vi "tm484_highcontrastmode.vi"() -> ()   [LabVIEW 2019]
panel:
  in  "High Contrast":bool
  out "Timestamp":dbl
  out "DCAM Version":string
  out "Library Version":string
  out "Image":u16[][](graph)
  out "Frames Per Second":dbl
  in  "Quit":bool
  out "Error Out":errorcluster {"code" format="%.0x"}
  # "This is just a simple example\nof how to capture and display\nlive data."
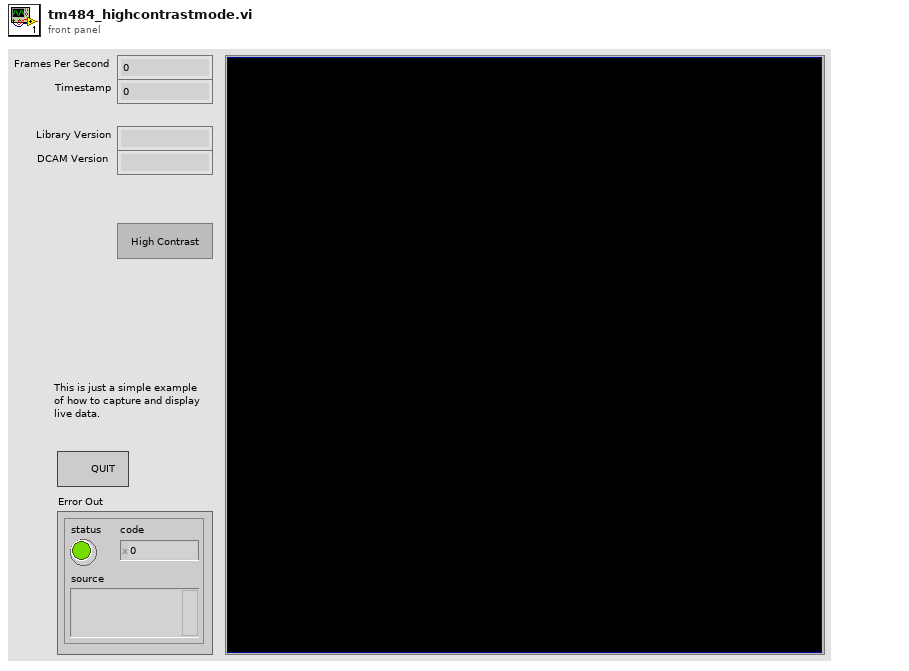
[diagram p1: front panel]
types:
  T1 = cluster{"Capture Library":string, "DCAM-API":string}
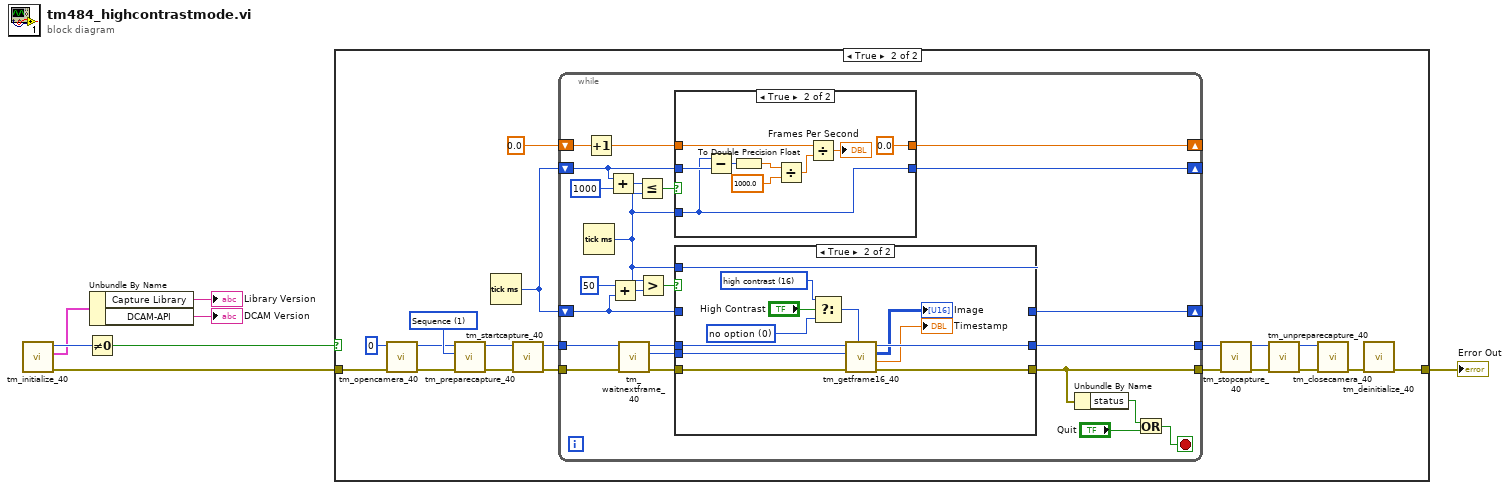
[diagram p0: block diagram]
diagram:
  n1 = call <userlib>:"tm_initialize_40.vi"() -> ("error out"=w4:errorcluster, "Version Info"=w3:T1, "Number Of Cameras"=w5:u32)  [unwired: 8 in, 1 out]
  n2 = Not Equal To 0?(x=w5) -> (x != 0?=w7:bool)
  n3 = Unbundle By Name(w3) -> ("Capture Library"=→"Library Version":string, "DCAM-API"=→"DCAM Version":string)
  n4 = case shown="True" w7 {
    tunnel: w4 -> [w8 w27]
    tunnel: [w8 w24] -> w6
    frame False {
    }
    frame True {
      w15 = 1 items=["Snap", "Sequence"] ("Capture mode")
      n5 = call <userlib>:"tm_opencamera_40.vi"("error in (no error)"=w27, "Camera Index"=u32 0) -> ("error out"=w9:errorcluster, "Handle out"=w10:u32)  [unwired: 7 in, 1 out]
      n6 = call <userlib>:"tm_preparecapture_40.vi"("error in (no error)"=w9, "Capture mode"=w15, "Handle in"=w10) -> ("error out"=w13:errorcluster, "Handle out"=w14:u32)  [unwired: 5 in, 2 out]
      n7 = Tick Count (ms)() -> (millisecond timer value=w11:u32)
      n8 = call <userlib>:"tm_startcapture_40.vi"("error in (no error)"=w13, "Handle in"=w14) -> ("error out"=w16:errorcluster, "Handle out"=w17:u32)  [unwired: 8 in]
      n9 = while {
        tunnel: [w30] -> w20
        tunnel: [w31] -> w21
        tunnel: w17 -> [w48]
        tunnel: w16 -> [w49]
        shift-right: [w46] -> _
        shift-left: w11 -> [w43]
        shift-right: [w47] -> _
        shift-left: 0.0 -> [w40]
        shift-right: [w29] -> _
        shift-left: w11 -> [w32]
        stop <- w28 stop-if-true
        n10 = Tick Count (ms)() -> (millisecond timer value=w33:u32)
        n11 = Increment(x=w40) -> (x+1=w41:dbl)
        n12 = Add(x=w43, y=u32 1000) -> (x+y=w45:u32)
        n13 = Add(x=u32 50, y=w32) -> (x+y=w35:u32)
        n14 = call <userlib>:"tm_waitnextframe_40.vi"("error in (no error)"=w49, "Handle in"=w48) -> ("error out"=w38:errorcluster, "Frame Index"=w37:i32, "Handle out"=w39:u32)  [unwired: 6 in, 1 out]
        n15 = Less Or Equal?(x=w45, y=w33) -> (x <= y?=w42:bool)
        n16 = Greater?(x=w33, y=w35) -> (0:w34:bool)
        n17 = case shown="True" w42 {
          tunnel: w43 -> [w68 w71]
          tunnel: [w68 w69] -> w46
          tunnel: w41 -> [w67 w75]
          tunnel: w33 -> [_ w69]
          tunnel: [w67 0.0] -> w47
          frame False {
          }
          frame True {
            n18 = Subtract(x=w69, y=w71) -> (x-y=w70:u32)
            n19 = To Double Precision Float(number=w70) -> (double precision float=w77:dbl)
            n20 = Divide(x=w77, y=1000.0) -> (x/y=w74:dbl)
            n21 = Divide(x=w75, y=w74) -> (x/y=→"Frames Per Second":dbl)
          }
        }
        n22 = case shown="True" w34 {
          tunnel: w39 -> [w54 w66]
          tunnel: w38 -> [w53 w65]
          tunnel: w37 -> [_ w59]
          tunnel: w32 -> [w52 _]
          tunnel: w33 -> [_ w64]
          tunnel: [w54 w62] -> w30
          tunnel: [w53 w63] -> w31
          tunnel: [w52 w64] -> w29
          frame False {
          }
          frame True {
            w56 = 0 items=["no option"=0, "high contrast"=16] ("Options")
            w57 = 16 items=["no option"=0, "high contrast"=16] ("Options")
            n23 = Select(t=w57, s="High Contrast", f=w56) -> (s? t:f=w58:i32)
            n24 = call <userlib>:"tm_getframe16_40.vi"("Options"=w58, "error in (no error)"=w65, "Frame Index"=w59, "Handle in"=w66) -> ("error out"=w63:errorcluster, "Timestamp"=→"Timestamp":dbl, "Data"=→"Image":u16[][], "Handle out"=w62:u32)  [unwired: 4 in]
          }
        }
        n25 = Unbundle By Name(w31) -> ("status"=w51:bool)
        n26 = Or(x=w51, y="Quit") -> (x .or. y?=w28:bool)
      }
      n27 = call <userlib>:"tm_stopcapture_40.vi"("error in (no error)"=w21, "Handle in"=w20) -> ("error out"=w18:errorcluster, "Handle out"=w19:u32)  [unwired: 8 in]
      n28 = call <userlib>:"tm_unpreparecapture_40.vi"("error in (no error)"=w18, "Handle in"=w19) -> ("error out"=w23:errorcluster, "Handle out"=w22:u32)  [unwired: 8 in]
      n29 = call <userlib>:"tm_closecamera_40.vi"("error in (no error)"=w23, "Handle in"=w22) -> ("error out"=w25:errorcluster)  [unwired: 9 in]
      n30 = call <userlib>:"tm_deinitialize_40.vi"("error in (no error)"=w25) -> ("error out"=w24:errorcluster)  [unwired: 10 in]
    }
  }
  "Error Out" <- w6
